vi "AddEvtModule.vi"(8 "Error In":errorcluster[](array[cluster]), 11 "Bus in":refnum<class "Bus.lvclass">) -> (0 "Error Out":errorcluster[](array[cluster]), 2 "clBroadcastEvents":T1, 3 "Bus out":refnum<class "Bus.lvclass">)   [LabVIEW 2014]
uses:
  Events/EventModule/Main.vi
  Events/EventModule/EventModule.lvlib
  <userlib>/NIST/NistModuleAdminLib/NistModuleAdmin/NistModuleAdmin.lvclass
  <userlib>/NIST/NISTErrorLib/NISTErrorLib.lvlib
  Bus.lvclass
  Events/EventModule/Protected/clEventType.ctl
  Events/EventModule/Protected/Broadcasts/clBroadcastEvents.ctl
panel:
  # "If you want to add other Broadcast Events, open this typedef, copy an existing event and rename it to your event name.\n\nNext create a typedef for the  data and put it into PublicAPI/Arguments/Broadcasts"
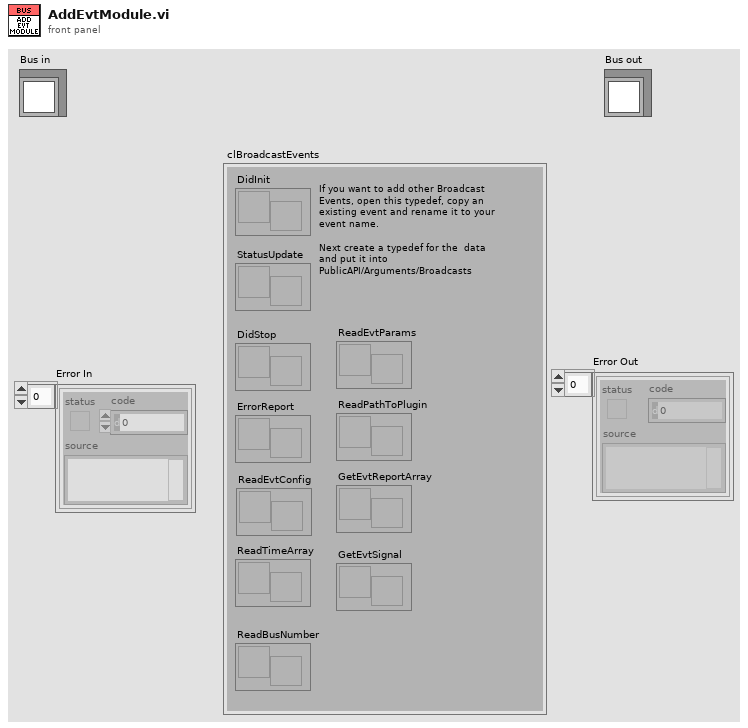
[diagram p1: front panel]
types:
  T1 = typedef "EventModule.lvlib/clBroadcastEvents.ctl" = cluster{"DidInit":refnum<user-event>, "StatusUpdate":refnum<user-event>, "ErrorReport":refnum<user-event>, "DidStop":refnum<user-event>, "ReadEvtConfig":refnum<user-event>, "ReadTimeArray":refnum<user-event>, "ReadEvtParams":refnum<user-event>, "GetEvtReportArray":refnum<user-event>, "ReadPathToPlugin":refnum<user-event>, "GetEvtSignal":refnum<user-event>, "ReadBusNumber":refnum<user-event>}
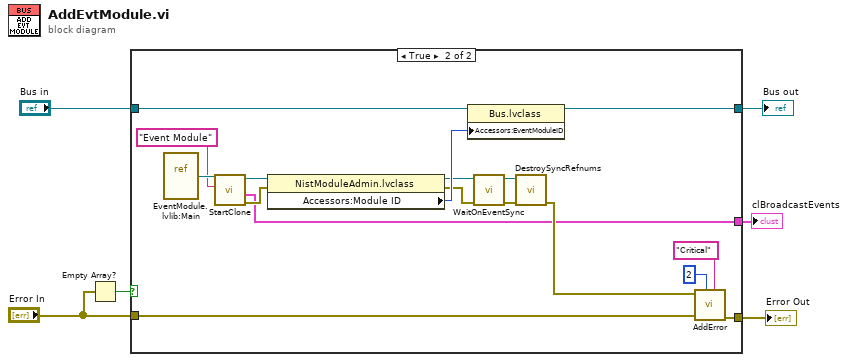
[diagram p0: block diagram]
diagram:
  n1 = Empty Array?(array="Error In") -> (empty?=w3:bool)
  n2 = case shown="True" w3 {
    tunnel: [w7 w14] -> w4
    tunnel: [w8 w20] -> w5
    tunnel: "Bus in" -> [w8 w25]
    tunnel: "Error In" -> [w7 w13]
    tunnel: [_ w9] -> w1
    frame False {
    }
    frame True {
      n3 = vi-ref "EventModule.lvlib:Main.vi"() -> (w24:refnum<vi>)
      n4 = call "StartClone.vi"("ModuleName"="Event Module", "VI Refnum"=w24) -> ("error out"=w21:errorcluster, "clBroadcastEvents"=w9:T1, "ModuleAdmin"=w22:refnum<class "NistModuleAdmin.lvclass">)  [unwired: 7 in]
      n5 = property class="NistModuleAdmin.lvclass"(reference=w22, error in=w21) -> (reference out=w17:refnum<class "NistModuleAdmin.lvclass">, error out=w18:errorcluster, "Accessors:Module ID"=w19:i32)
      n6 = property class="Bus.lvclass"(reference=w25, "Accessors:EventModuleID"=w19) -> (reference out=w20:refnum<class "Bus.lvclass">)  [unwired: 1 in, 1 out]
      n7 = call <userlib>:"WaitOnEventSync.vi"("error in (no error)"=w18, "ModuleAdmin"=w17) -> ("error out"=w16:errorcluster, "ModuleAdmin"=w15:refnum<class "NistModuleAdmin.lvclass">)  [unwired: 8 in]
      n8 = call <userlib>:"DestroySyncRefnums.vi"("error in (no error)"=w16, "ModuleAdmin"=w15) -> ("error out"=w10:errorcluster)  [unwired: 9 in]
      n9 = call <userlib>:"AddError.vi"("Severity"="Critical", "Priority"=u8 2, "ErrorArray"=w13, "error in (no error)"=w10) -> ("ErrorArray"=w14:errorcluster[])  [unwired: 6 in, 1 out]
    }
  }
  "Bus out" <- w5
  "Error Out" <- w4
  "clBroadcastEvents" <- w1
